vi "adjustAngle_06.vi"() -> ()   [LabVIEW 2011]
panel:
  in  "Motion":u16(ring) items=["direct", "positive", "negative"]
  in  "first":bool=TRUE
  out "tStart":dbl
  in  "time done (s)":dbl
  in  "Reverse delay (s)":dbl=2.0
  out "Wait to set":bool
  out "IO error":errorcluster
  in  "stop":bool
  out "Angle Indicator (deg)":dbl=20.6 caption="Angle (deg)" format="%.1f"
  in  "Angle (deg)":dbl format="%.1f"
  out "P (torr)":dbl=19.959999999999997 format="%.2f"
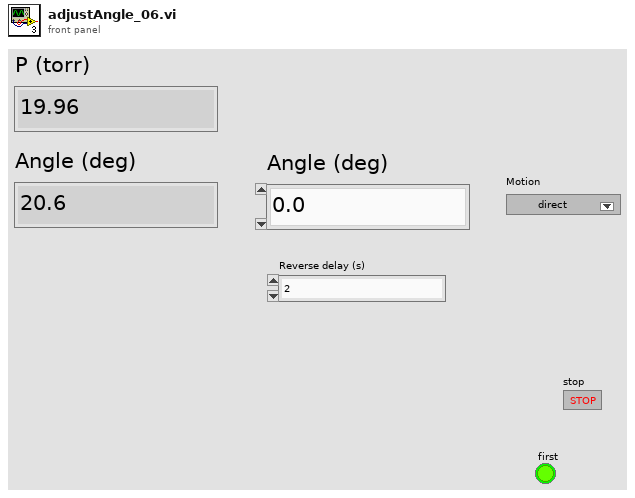
[diagram p1: front panel]
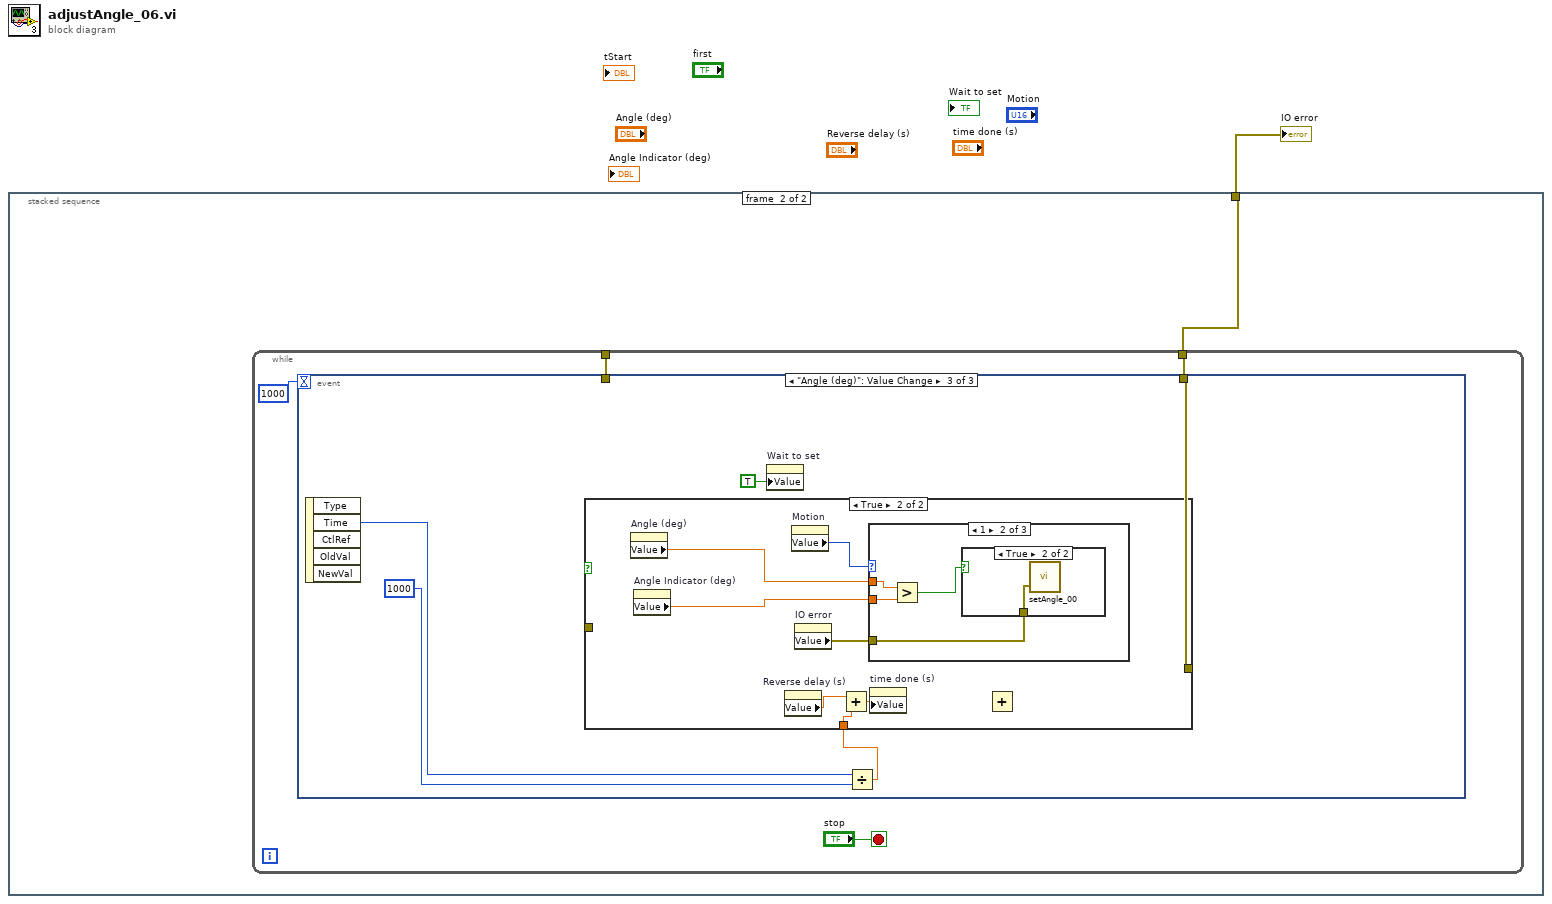
[diagram p0: block diagram]
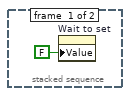
[diagram p2: hidden frame]
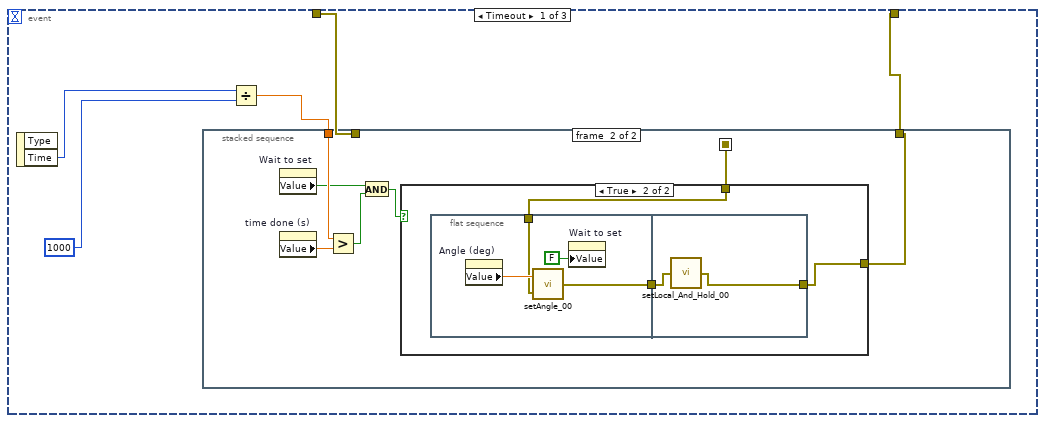
[diagram p3: hidden frame]
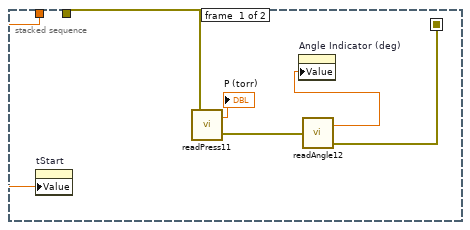
[diagram p4: hidden frame]
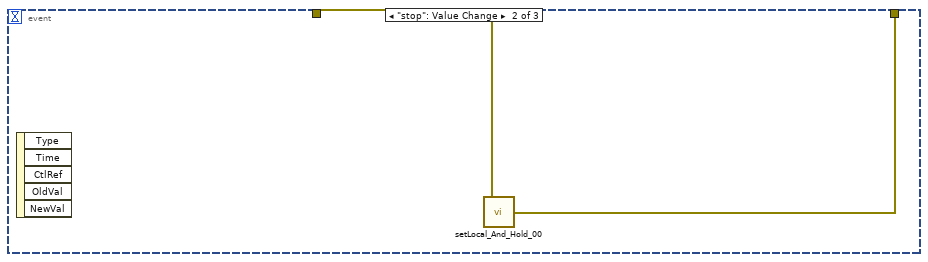
[diagram p6: hidden frame]
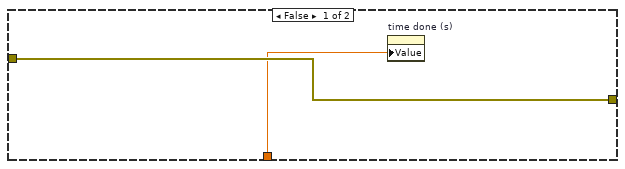
[diagram p7: hidden frame]
diagram:
  n1 = stacked-sequence {
    tunnel: [_ w3] -> w1
    frame #0 {
      n2 = property on="Wait to set" class="Bool (strict)"("Value"=FALSE ("Wait to set")) -> ()  [unwired: 2 in, 2 out]
    }
    frame #1 {
      n3 = while {
        tunnel: [w7] -> w4
        tunnel: [w6] -> w3
        stop <- "stop" stop-if-true
        n4 = event shown="[2] \"Angle (deg)\": Value Change" {
          selector: _ -> [_ _ _]
          dyn-events: _ -> [_ _ _]
          timeout: 1000 -> [_ _ _]
          tunnel: w7 -> [w13 w38 _]
          tunnel: [w12 w37 w43] -> w6
          event Timeout {
            n5 = event-data() -> ("Time"=w11:u32)  [unwired: 1 in, 1 out]
            n6 = Divide(x=w11, y=u32 1000) -> (x/y=w9:dbl)
            n7 = stacked-sequence {
              seq-local: [w16 _] -> [_ w20]
              tunnel: w13 -> [w19 _]
              tunnel: w9 -> [w15 w26]
              tunnel: [_ w22] -> w12
              frame #0 {
                n8 = property on="tStart" class="DigNum (strict)"("Value"=w15) -> ()  [unwired: 2 in, 2 out]
                n9 = call "readPress11.vi"("error in"=w19) -> ("P"=→"P (torr)":dbl, "error out"=w17:errorcluster)
                n10 = call "readAngle12.vi"("error in"=w17) -> ("angle"=w14:dbl, "error out"=w16:errorcluster)
                n11 = property on="Angle Indicator (deg)" class="DigNum (strict)"("Value"=w14) -> ()  [unwired: 2 in, 2 out]
              }
              frame #1 {
                n12 = property on="Wait to set" class="Bool (strict)"() -> ("Value"=w21:bool)  [unwired: 2 in, 2 out]
                n13 = property on="time done (s)" class="DigNum (strict)"() -> ("Value"=w25:dbl)  [unwired: 2 in, 2 out]
                n14 = Greater?(x=w26, y=w25) -> (0:w24:bool)
                n15 = And(x=w21, y=w24) -> (x .and. y?=w23:bool)
                n16 = case shown="True" w23 {
                  tunnel: [w27 w30] -> w22
                  tunnel: w20 -> [w27 w28]
                  frame False {
                  }
                  frame True {
                    n17 = flat-sequence {
                      tunnel: [w33] -> w29
                      tunnel: w28 -> [w31]
                      tunnel: [w35] -> w30
                      tunnel: w29 -> [w36]
                      frame #0 {
                        n18 = property on="Angle (deg)" class="DigNum (strict)"() -> ("Value"=w34:dbl)  [unwired: 2 in, 2 out]
                        n19 = call "setAngle_00.vi"("error in (no error)"=w31, "Angle (deg)"=w34) -> ("error out"=w33:errorcluster)
                        n20 = property on="Wait to set" class="Bool (strict)"("Value"=FALSE ("Wait to set")) -> ()  [unwired: 2 in, 2 out]
                      }
                      frame #1 {
                        n21 = call "setLocal_And_Hold_00.vi"("error in (no error)"=w36) -> ("error out"=w35:errorcluster)
                      }
                    }
                  }
                }
              }
            }
          }
          event "stop": Value Change {
            n22 = event-data() -> ()  [unwired: 1 in, 5 out]
            n23 = call "setLocal_And_Hold_00.vi"("error in (no error)"=w38) -> ("error out"=w37:errorcluster)
          }
          event "Angle (deg)": Value Change {
            n24 = event-data() -> ("Time"=w42:u32)  [unwired: 1 in, 4 out]
            n25 = property on="Wait to set" class="Bool (strict)"("Value"=TRUE ("Wait to set")) -> ()  [unwired: 2 in, 2 out]
            n26 = Divide(x=w42, y=u32 1000) -> (x/y=w40:dbl)
            n27 = case shown="True" {
              selector: _ -> [_ _]
              tunnel: _ -> [w45 _]
              tunnel: [w45 _] -> w43
              tunnel: w40 -> [w44 w50]
              frame False {
                n28 = property on="time done (s)" class="DigNum (strict)"("Value"=w44) -> ()  [unwired: 2 in, 2 out]
              }
              frame True {
                n29 = property on="Angle (deg)" class="DigNum (strict)"() -> ("Value"=w47:dbl)  [unwired: 2 in, 2 out]
                n30 = property on="Angle Indicator (deg)" class="DigNum (strict)"() -> ("Value"=w46:dbl)  [unwired: 2 in, 2 out]
                n31 = property on="Reverse delay (s)" class="DigNum (strict)"() -> ("Value"=w51:dbl)  [unwired: 2 in, 2 out]
                n32 = property on="Motion" class="Ring (strict)"() -> ("Value"=w49:u16)  [unwired: 2 in, 2 out]
                n33 = property on="IO error" class="Clust (strict)"() -> ("Value"=w48:errorcluster)  [unwired: 2 in, 2 out]
                n34 = Add(x=w51, y=w50) -> (x+y=w52:dbl)
                n35 = case shown="1" w49 {
                  tunnel: w48 -> [_ w56 _]
                  tunnel: w47 -> [_ w55 _]
                  tunnel: w46 -> [_ w54 _]
                  frame 0, Default {
                  }
                  frame 1 {
                    n36 = Greater?(x=w55, y=w54) -> (0:w53:bool)
                    n37 = case shown="True" w53 {
                      tunnel: w56 -> [_ w57]
                      frame False {
                      }
                      frame True {
                        n38 = call "setAngle_00.vi"("error in (no error)"=w57) -> ()  [unwired: 1 in, 1 out]
                      }
                    }
                  }
                  frame 2 {
                  }
                }
                n39 = property on="time done (s)" class="DigNum (strict)"("Value"=w52) -> ()  [unwired: 2 in, 2 out]
                n40 = Add() -> ()  [unwired: 2 in, 1 out]
              }
            }
          }
        }
      }
    }
  }
  "IO error" <- w1
